vi "split2.vi"(4 "error in":errorcluster, 5 "Waveforms":waveform(i16)[](array[waveform]), 7 "full file path":path) -> (0 "error out":errorcluster, 1 "compressed":cluster{"appended path":path, waveform(i16)[]}, 2 "first":cluster{"appended path":path, waveform(i16)[]})   [LabVIEW 2010]
uses:
  <vilib>/Waveform/WDTOps.llb/WDT Get Waveform Subset I16.vi
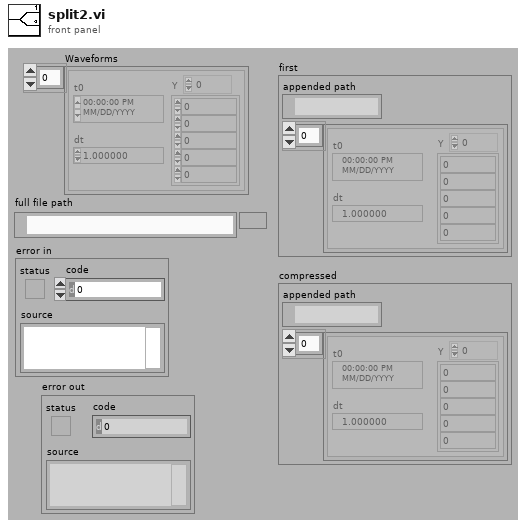
[diagram p1: front panel]
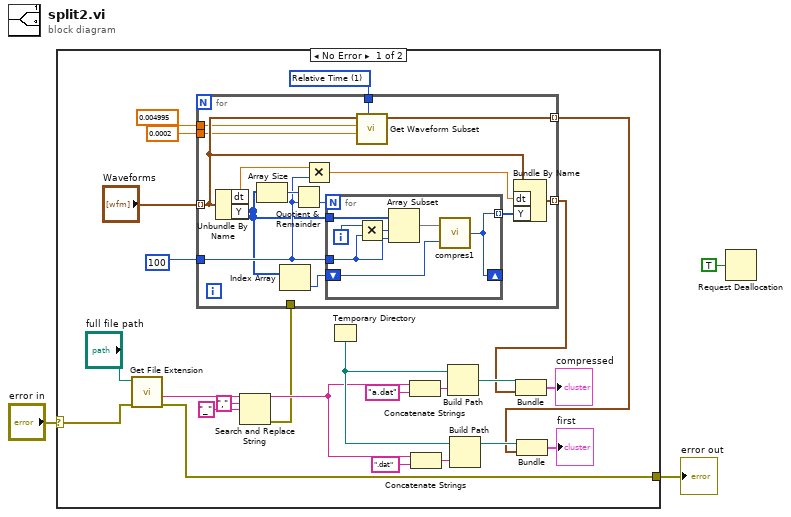
[diagram p0: block diagram]
diagram:
  n1 = case shown="No Error" "error in" {
    selector: "error in" -> [w5 w49]
    tunnel: [w4 w49] -> w2
    frame No Error {
      w25 = u16 1 items=["Index", "Relative Time"] ("start/duration format")
      n2 = call <vilib>:"Get File Extension.vi"("error in (no error)"=w5, "file"="full file path") -> ("error out"=w4:errorcluster, "filename without extension"=w10:string)  [unwired: 6 in, 2 out]
      n3 = Search and Replace String(input string=w10, search string=",", replace string="_" ("replace string (\"\")")) -> (result string=w9:string, error out=w6:errorcluster)  [unwired: 5 in, 2 out]
      n4 = for {
        tunnel: "Waveforms" -> [w34] mode=indexing
        tunnel: [w36] -> w14 mode=indexing
        tunnel: 100 -> [w35]
        tunnel: w25 -> [w33]
        tunnel: 0.004995 ("duration") -> [w32]
        tunnel: 0.0002 ("duration") -> [w31]
        tunnel: [w30] -> w13 mode=indexing
        tunnel: w6 -> [_]
        n5 = Unbundle By Name(w34) -> ("dt"=w38:dbl, "Y"=w29:i16[])
        n6 = Array Size(array=w29) -> (size(s)=w41:i32)
        n7 = Index Array(array=w29) -> (element=w28:i16)  [unwired: 1 in]
        n8 = Quotient & Remainder(x=w41, y=w35) -> (floor(x/y)=w40:i32)  [unwired: 1 out]
        n9 = Multiply(x=w38, y=w35) -> (x*y=w37:dbl)
        n10 = for {
          N: w40 -> [_]
          tunnel: w29 -> [w48]
          tunnel: w35 -> [w45]
          tunnel: [w43] -> w39 mode=indexing
          shift-right: [w43] -> _
          shift-left: w28 -> [w42]
          i -> [w44]
          n11 = Multiply(x=w44, y=w45) -> (x*y=w46:i32)
          n12 = Array Subset(array=w48, index=w46, length=w45) -> (w47:i16[])
          n13 = call "compres1.vi"("Numeric"=w42, "Array"=w47) -> ("Numeric 2"=w43:i16)
        }
        n14 = call-poly <vilib>:"Get Waveform Subset.vi"("start/duration format"=w33, "duration"=w31, "start samples/time"=w32, "waveform in"=w34) -> ("waveform out"=w30:waveform(i16))  [unwired: 2 in, 3 out]
        n15 = Bundle By Name(cluster=w34, "dt"=w37, "Y"=w39) -> (w36:waveform(i16))
      }
      n16 = Temporary Directory() -> (w22:path)
      n17 = Concatenate Strings(w9, "a.dat" ("name or relative path")) -> (w18:string)
      n18 = Concatenate Strings(w9, ".dat" ("search string")) -> (w19:string)
      n19 = Build Path(base path=w22, name or relative path=w18) -> (appended path=w16:path)
      n20 = Build Path(base path=w22, name or relative path=w19) -> (appended path=w17:path)
      n21 = Bundle("appended path"=w16, w14) -> (→"compressed":cluster{"appended path":path, waveform(i16)[]})  [unwired: 1 in]
      n22 = Bundle("appended path"=w17, w13) -> (→"first":cluster{"appended path":path, waveform(i16)[]})  [unwired: 1 in]
    }
    frame Error {
    }
  }
  "error out" <- w2
  n23 = Request Deallocation(TRUE ("flag")) -> ()
